vi "knownhosts_readline.vi"() -> ()   [LabVIEW 2013]
doc: "Illustrates how to read known hosts from a multi-line string."
uses:
  libssh2/libssh2_knownhost.ctl
  libssh2/Known Host Refnum.ctl
  libssh2/libssh2_init_default.vi
  libssh2/libssh2.lvlib
panel:
  out "error out":errorcluster
  out "known hosts":T1[](array[typedef])
  in  "lines":string="git.code.sf.net ssh-ed25519 AAAAC3NzaC1lZDI1NTE5AAAAIGObtXLh/mZom0pXjE5Mu211O+JvtzolqdNKVA+XJ466\ngit.code.sf.net ssh-rsa AAAAB3NzaC1yc2EAAAABIwAAAQEAoMesJ60dow5VqNsIqIQMBNmSYz6txSC5YSUXzPNWV4VIWTWdqbQoQuIu+oYGhBMoeaSWWCiVIDTwFDzQXrq8CwmyxWp+2TTuscKiOw830N2ycIVmm3ha0x6VpRGm37yo+z+bkQS3m/sE7bkfTU72GbeKufFHSv1VLnVy9nmJKFOraeKSHP/kjmatj9aC7Q2n8QzFWWjzMxVGg79TUs7sjm5KrtytbxfbLbKtrkn8OXsRy1ib9hKgOwg+"
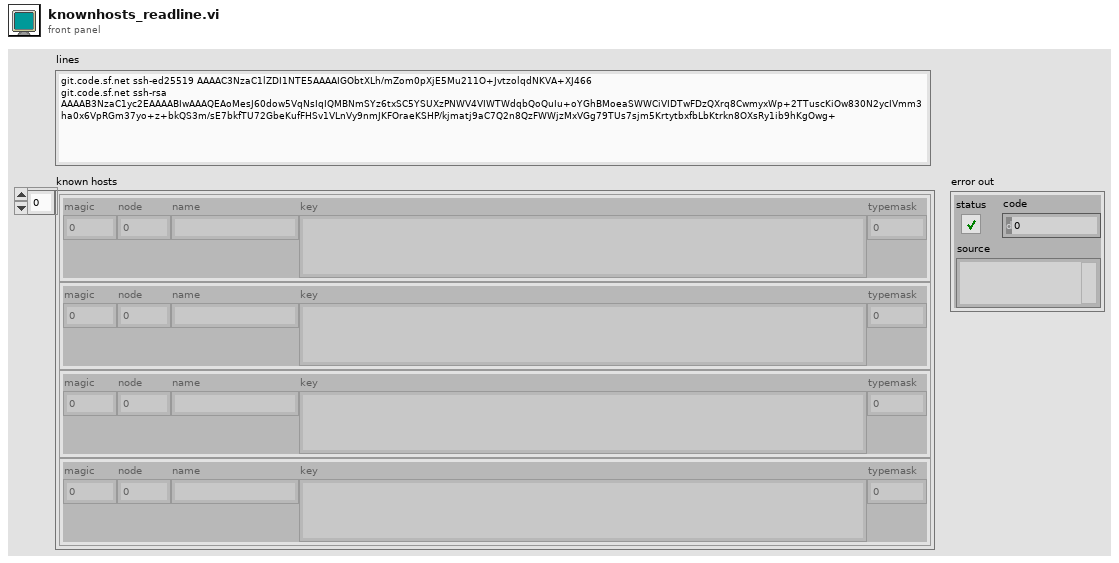
[diagram p1: front panel]
types:
  T1 = typedef "libssh2.lvlib/libssh2_knownhost.ctl" = cluster{"magic":u32, "node":u64, "name":string, "key":string, "typemask":i32}
  T2 = typedef "libssh2.lvlib/Known Host Refnum.ctl" = refnum<k1>
  T3 = typedef "libssh2.lvlib/Session Refnum.ctl" = refnum<k1>
  T4 = typedef "libssh2.lvlib/Known Host Collection Refnum.ctl" = refnum<k1>
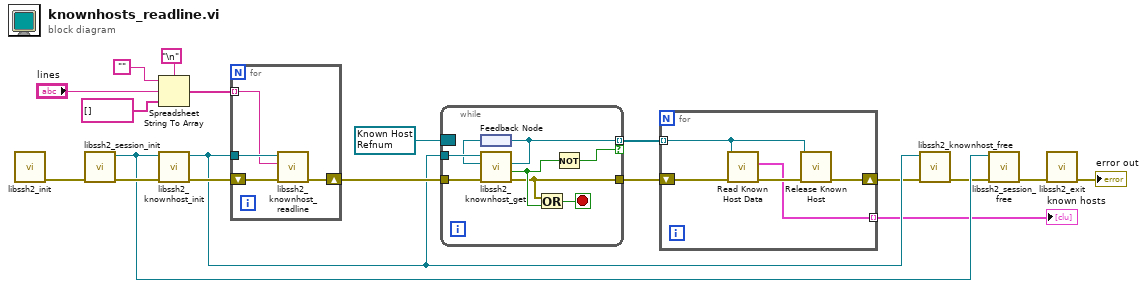
[diagram p0: block diagram]
diagram:
  w9 = T2 refnum items=["Host"] ("next")
  n1 = call-poly "libssh2_init.vi"() -> ("error out"=w19:errorcluster)  [unwired: 11 in]
  n2 = call "libssh2_session_init.vi"("error in (no error)"=w19) -> ("error out"=w18:errorcluster, "session"=w17:T3)  [unwired: 9 in]
  n3 = Spreadsheet String To Array(delimiter (Tab)="\n", format string="", spreadsheet string="lines", array type (2D Dbl)=string[] []) -> (array=w6:string[])
  n4 = call "libssh2_knownhost_init.vi"("error in (no error)"=w18, "session"=w17) -> ("error out"=w14:errorcluster, "known hosts collection"=w12:T4)  [unwired: 8 in]
  n5 = for {
    tunnel: w12 -> [w21]
    tunnel: w6 -> [w20] mode=indexing
    shift-right: [w22] -> w13
    shift-left: w14 -> [w23]
    n6 = call "libssh2_knownhost_readline.vi"("error in (no error)"=w23, "line"=w20, "known hosts collection"=w21) -> ("error out"=w22:errorcluster)  [unwired: 8 in]
  }
  n7 = while {
    tunnel: w13 -> [w31]
    tunnel: [w25] -> w11
    tunnel: w12 -> [w30]
    border: w9 -> [_]
    tunnel: [w27] -> w8 mode=indexing if=w24
    stop <- w29 stop-if-true
    n8 = feedback #1() -> (w28:T2)
    n9 = call "libssh2_knownhost_get.vi"("error in (no error)"=w31, "previous"=w28, "known hosts collection"=w30) -> ("error out"=w25:errorcluster, "end reached"=w26:bool, "next"=w27:T2)  [unwired: 6 in]
    n10 = feedback-in #1(w27) -> ()
    n11 = Or(x=w25, y=w26) -> (x .or. y?=w29:bool)
    n12 = Not(x=w26) -> (.not. x?=w24:bool)
  }
  n13 = for {
    shift-right: [w36] -> w10
    shift-left: w11 -> [w35]
    tunnel: w8 -> [w32] mode=indexing
    tunnel: [w33] -> w2 mode=indexing
    n14 = call "Read Known Host Data.vi"("error in (no error)"=w35, "known host"=w32) -> ("error out"=w34:errorcluster, "known host data"=w33:T1)  [unwired: 8 in]
    n15 = call "Release Known Host.vi"("error in (no error)"=w34, "known host"=w32) -> ("error out"=w36:errorcluster)  [unwired: 9 in]
  }
  "known hosts" <- w2
  n16 = call "libssh2_knownhost_free.vi"("error in (no error)"=w10, "known hosts collection"=w12) -> ("error out"=w16:errorcluster)  [unwired: 9 in]
  n17 = call "libssh2_session_free.vi"("error in (no error)"=w16, "session"=w17) -> ("error out"=w15:errorcluster)  [unwired: 9 in]
  n18 = call "libssh2_exit.vi"("error in (no error)"=w15) -> ("error out"=→"error out":errorcluster)  [unwired: 10 in]
